vi "HIOKI PW3390 Conf ZeroSp.vi"(0 "VISA Resource":refnum<visa-resource-name>, 1 "Set/Query (F: Set)":bool, 5 "Zero suppress (0: OFF)":enum16{"OFF", "0.1%f.s.", "0.5%f.s."}(ring), 11 "error in (no error)":errorcluster, 12 "OPC query (T: ON)":bool=TRUE, 13 "Error Out (F: Off)":bool) -> (4 "VISA Resource out":refnum<visa-resource-name>, 6 "Zero suppress out":enum16{"OFF", "0.1%f.s.", "0.5%f.s."}(ring), 15 "error out":errorcluster)   [LabVIEW 2009]
doc: "Set/Query\n Set: Send the setting commands for the device.\n Query: Query the setting of the device.\n\nZero Suppress\n Sets the Zero Suppress."
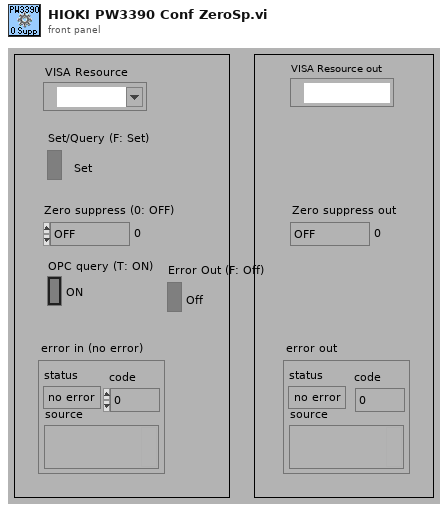
[diagram p1: front panel]
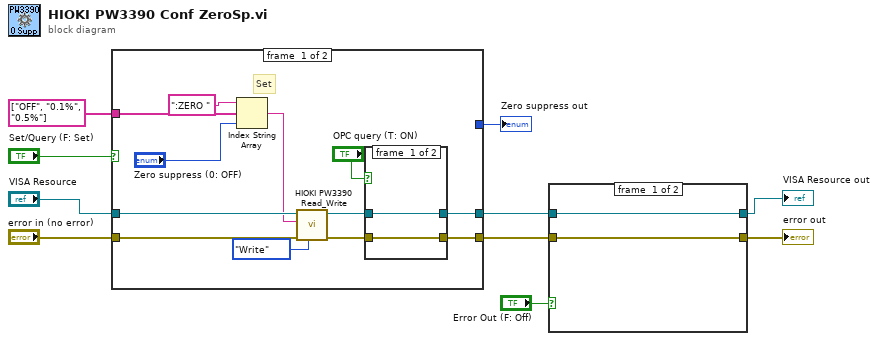
[diagram p0: block diagram]
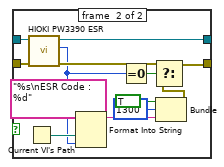
[diagram p2: hidden frame]
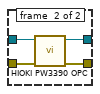
[diagram p3: hidden frame]
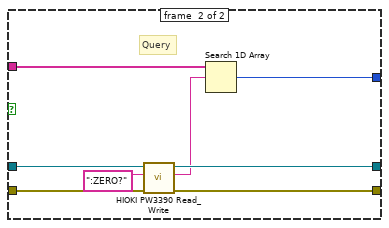
[diagram p4: hidden frame]
diagram:
  n1 = case shown="FALSE" "Set/Query (F: Set)" {
    tunnel: "error in (no error)" -> [w21 w35]
    tunnel: [w11 w32] -> w7
    tunnel: "VISA Resource" -> [w22 w34]
    tunnel: [w12 w33] -> w6
    tunnel: [_ w30] -> w4
    tunnel: string[] ["OFF", "0.1%", "0.5%"] ("Strings []") -> [w17 w29]
    frame #0 {
      # "Set"
      n2 = Index String Array(1:"Zero suppress (0: OFF)", 2:w17, 3:":ZERO ") -> (0:w16:string)
      n3 = call <instrlib>:"HIOKI PW3390 Read_Write.vi"("Read/Write"=enum16{"Read", "Write"}."Write", "error in (no error)"=w21, "data in"=w16, "VISA Resource"=w22) -> ("error out"=w13:errorcluster, "VISA Resource out"=w14:refnum<visa-resource-name>)  [unwired: 5 in, 1 out]
      n4 = case shown="TRUE" "OPC query (T: ON)" {
        tunnel: [w24 w28] -> w12
        tunnel: [w23 w27] -> w11
        tunnel: w14 -> [w24 w26]
        tunnel: w13 -> [w23 w25]
        frame #0 {
        }
        frame #1 {
          n5 = call <instrlib>:"HIOKI PW3390 OPC.vi"("error in (no error)"=w25, "VISA Resource"=w26) -> ("error out"=w27:errorcluster, "VISA Resource out"=w28:refnum<visa-resource-name>)  [unwired: 7 in, 1 out]
        }
      }
    }
    frame #1 {
      # "Query"
      n6 = call <instrlib>:"HIOKI PW3390 Read_Write.vi"("error in (no error)"=w35, "data in"=":ZERO?", "VISA Resource"=w34) -> ("error out"=w32:errorcluster, "data out"=w31:string, "VISA Resource out"=w33:refnum<visa-resource-name>)  [unwired: 6 in]
      n7 = Search 1D Array(1D array=w29, element=w31) -> (index of element=w30:i32)  [unwired: 1 in]
    }
  }
  "Zero suppress out" <- w4
  n8 = case shown="TRUE" "Error Out (F: Off)" {
    tunnel: w6 -> [w38 w51]
    tunnel: w7 -> [w37 w50]
    tunnel: [w37 w40] -> w5
    tunnel: [w38 w49] -> w1
    frame #0 {
    }
    frame #1 {
      n9 = Current VI's Path() -> (path=w47:path)
      n10 = call <instrlib>:"HIOKI PW3390 ESR.vi"("error in (no error)"=w50, "VISA Resource"=w51) -> ("error out"=w41:errorcluster, "Output Value"=w39:u8, "VISA Resource out"=w49:refnum<visa-resource-name>)  [unwired: 6 in, 1 out]
      n11 = Format Into String(format string="%s\nESR Code : %d", w47, w39) -> (resulting string=w43:string)  [unwired: 2 in, 1 out]
      n12 = Equal To 0?(x=w39) -> (x = 0?=w48:bool)
      n13 = Bundle("status"=TRUE, "code"=1300, w43) -> (w42:cluster{"status":bool, "code":i32, string})  [unwired: 1 in]
      n14 = Select(t=w41, s=w48, f=w42) -> (s? t:f=w40:errorcluster)
    }
  }
  "error out" <- w5
  "VISA Resource out" <- w1
